vi "rsscope_core_global.vi"() -> ()   [LabVIEW 2014] (continued)
"Supported Models"="", "Instrument Options"="", "Flags"=0, "Help"="Starts the measurement.\n\nAvailable Repeated Capabilities:\nNone\n\nRemote-control command(s):\nPOWer:DONRes:EXECute"}, {"Level"=3, "Class Only"=FALSE, "Identifier"="RSSCOPE_ATTR_POWER_DYNAMIC_ON_RESISTANCE_AVERAGE", "Descriptive Name"="Power Dynamic On Resistance Average", "Data Type"=3, "Command"="POW:DONR:AVG", "Access"=2, "Range Table"="", "Read Callback"="", "Write Callback"="", "Supported Models"="", "Instrument Options"="", "Flags"=0, "Help"="Enables/disables averaging.\n\nAvailable Repeated Capabilities:\nNone\n\nRemote-control command(s):\nPOWer:DONRes:AVG"}, {"Level"=3, "Class Only"=FALSE, "Identifier"="RSSCOPE_ATTR_POWER_DYNAMIC_ON_RESISTANCE_SCALING", "Descriptive Name"="Power Dynamic On Resistance Scaling", "Data Type"=0, "Command"="POW:DONR:AUTO", "Access"=2, "Range Table"="RsScope_rngPowerScaling", "Read Callback"="", "Write Callback"="", "Supported Models"="", "Instrument Options"="", "Flags"=0, "Help"="Selects the scaling for the display of the results.\n\nAvailable Repeated Capabilities:\nNone\n\nRemote-control command(s):\nPOWer:DONRes:AUTO"}, {"Level"=3, "Class Only"=FALSE, "Identifier"="RSSCOPE_ATTR_POWER_DYNAMIC_ON_RESISTANCE_ADD", "Descriptive Name"="Power Dynamic On Resistance Add To Report", "Data Type"=4, "Command"="POW:DONR:REP:ADD", "Access"=1, "Range Table"="", "Read Callback"="", "Write Callback"="", "Supported Models"="", "Instrument Options"="", "Flags"=0, "Help"="Adds the result to the report list.\n\nAvailable Repeated Capabilities:\nNone\n\nRemote-control command(s):\nPOWer:DONRes:REPort:ADD"}, {"Level"=3, "Class Only"=TRUE, "Identifier"="", "Descriptive Name"="Gate", "Data Type"=0, "Command"="", "Access"=0, "Range Table"="", "Read Callback"="", "Write Callback"="", "Supported Models"="", "Instrument Options"="", "Flags"=0, "Help"="Attributes with gate repeated capability."}, {"Level"=4, "Class Only"=FALSE, "Identifier"="RSSCOPE_ATTR_POWER_DYNAMIC_ON_RESISTANCE_GATE_START", "Descriptive Name"="Power Dynamic On Resistance Gate Start", "Data Type"=1, "Command"="POW:DONR:GATE{Gate}:START", "Access"=2, "Range Table"="", "Read Callback"="", "Write Callback"="", "Supported Models"="", "Instrument Options"="", "Flags"=0, "Help"="Start of the gate.\n\nAvailable Repeated Capabilities:\nGate: Gate1, Gate2, Gate3, Gate4, Gate5\r\n\nRemote-control command(s):\nPOWer:DONRes:GATE<m>:STARt"}, {"Level"=4, "Class Only"=FALSE, "Identifier"="RSSCOPE_ATTR_POWER_DYNAMIC_ON_RESISTANCE_GATE_STOP", "Descriptive Name"="Power Dynamic On Resistance Gate Stop", "Data Type"=1, "Command"="POW:DONR:GATE{Gate}:STOP", "Access"=2, "Range Table"="", "Read Callback"="", "Write Callback"="", "Supported Models"="", "Instrument Options"="", "Flags"=0, "Help"="Stop of the gate.\n\nAvailable Repeated Capabilities:\nGate: Gate1, Gate2, Gate3, Gate4, Gate5\r\n\nRemote-control command(s):\nPOWer:DONRes:GATE<m>STOP"}, {"Level"=3, "Class Only"=TRUE, "Identifier"="", "Descriptive Name"="Results", "Data Type"=0, "Command"="", "Access"=0, "Range Table"="", "Read Callback"="", "Write Callback"="", "Supported Models"="", "Instrument Options"="", "Flags"=0, "Help"="Results of dynamic on resistance measurement"}, {"Level"=4, "Class Only"=FALSE, "Identifier"="RSSCOPE_ATTR_POWER_DYNAMIC_ON_RESISTANCE_RESULT", "Descriptive Name"="Power Dynamic On Resistance Result", "Data Type"=1, "Command"="POW:DONR:RES:RES?", "Access"=0, "Range Table"="", "Read Callback"="", "Write Callback"="", "Supported Models"="", "Instrument Options"="", "Flags"=0, "Help"="Returns the result of the measurement\n\nAvailable Repeated Capabilities:\nNone\n\nRemote-control command(s):\nPOWer:DONRes:RESult:RESistance?"}, {"Level"=2, "Class Only"=TRUE, "Identifier"="", "Descriptive Name"="Efficiency", "Data Type"=0, "Command"="", "Access"=0, "Range Table"="", "Read Callback"="", "Write Callback"="", "Supported Models"="", "Instrument Options"="", "Flags"=0, "Help"="Power efficiency measurement."}, {"Level"=3, "Class Only"=FALSE, "Identifier"="RSSCOPE_ATTR_START_POWER_EFFICIENCY_MEASUREMENT", "Descriptive Name"="Start Power Efficiency Measurement", "Data Type"=4, "Command"="POW:EFF:EXEC", "Access"=1, "Range Table"="", "Read Callback"="", "Write Callback"="", "Supported Models"="", "Instrument Options"="", "Flags"=0, "Help"="Starts the measurement.\n\nAvailable Repeated Capabilities:\nNone\n\nRemote-control command(s):\nPOWer:EFFiciency:EXECute"}, {"Level"=3, "Class Only"=FALSE, "Identifier"="RSSCOPE_ATTR_POWER_EFFICIENCY_SCALING", "Descriptive Name"="Power Efficiency Scaling", "Data Type"=0, "Command"="POW:EFF:AUTO", "Access"=2, "Range Table"="RsScope_rngPowerScaling", "Read Callback"="", "Write Callback"="", "Supported Models"="", "Instrument Options"="", "Flags"=0, "Help"="Selects the scaling for the display of the results.\n\nAvailable Repeated Capabilities:\nNone\n\nRemote-control command(s):\nPOWer:EFFiciency:AUTO"}, {"Level"=3, "Class Only"=FALSE, "Identifier"="RSSCOPE_ATTR_POWER_EFFICIENCY_ADD", "Descriptive Name"="Power Efficiency Add To Report", "Data Type"=4, "Command"="POW:EFF:REP:ADD", "Access"=1, "Range Table"="", "Read Callback"="", "Write Callback"="", "Supported Models"="", "Instrument Options"="", "Flags"=0, "Help"="Adds the result to the report list.\n\nAvailable Repeated Capabilities:\nNone\n\nRemote-control command(s):\nPOWer:EFFiciency:REPort:ADD"}, {"Level"=3, "Class Only"=TRUE, "Identifier"="", "Descriptive Name"="Results", "Data Type"=0, "Command"="", "Access"=0, "Range Table"="", "Read Callback"="", "Write Callback"="", "Supported Models"="", "Instrument Options"="", "Flags"=0, "Help"="Results of the measurement."}, {"Level"=2, "Class Only"=TRUE, "Identifier"="", "Descriptive Name"="Switchingloss", "Data Type"=0, "Command"="", "Access"=0, "Range Table"="", "Read Callback"="", "Write Callback"="", "Supported Models"="", "Instrument Options"="", "Flags"=0, "Help"="Switchingloss measurement"}, {"Level"=3, "Class Only"=FALSE, "Identifier"="RSSCOPE_ATTR_START_POWER_SWITCHINGLOSS_MEASUREMENT", "Descriptive Name"="Start Power Switchingloss Measurement", "Data Type"=4, "Command"="POW:SWIT:EXEC", "Access"=1, "Range Table"="", "Read Callback"="", "Write Callback"="", "Supported Models"="", "Instrument Options"="", "Flags"=0, "Help"="Starts the measurement.\n\nAvailable Repeated Capabilities:\nNone\n\nRemote-control command(s):\nPOWer:SWITching:EXECute"}, {"Level"=3, "Class Only"=FALSE, "Identifier"="RSSCOPE_ATTR_POWER_SWITCHINGLOSS_TON_STATE", "Descriptive Name"="Power Switchingloss Turn On State", "Data Type"=3, "Command"="POW:SWIT:TON", "Access"=2, "Range Table"="", "Read Callback"="", "Write Callback"="", "Supported Models"="", "Instrument Options"="", "Flags"=0, "Help"="Enables the measurement during the Turn On period.\n\nAvailable Repeated Capabilities:\nNone\n\nRemote-control command(s):\nPOWer:SWITching:TON"}, {"Level"=3, "Class Only"=FALSE, "Identifier"="RSSCOPE_ATTR_POWER_SWITCHINGLOSS_TOF_STATE", "Descriptive Name"="Power Switchingloss Turn Off State", "Data Type"=3, "Command"="POW:SWIT:TOFF", "Access"=2, "Range Table"="", "Read Callback"="", "Write Callback"="", "Supported Models"="", "Instrument Options"="", "Flags"=0, "Help"="Enables the measurement during the Turn Off period.\n\nAvailable Repeated Capabilities:\nNone\n\nRemote-control command(s):\nPOWer:SWITching:TOFF"}, {"Level"=3, "Class Only"=FALSE, "Identifier"="RSSCOPE_ATTR_POWER_SWITCHINGLOSS_CONDUCTION_STATE", "Descriptive Name"="Power Switchingloss Conduction State", "Data Type"=3, "Command"="POW:SWIT:COND", "Access"=2, "Range Table"="", "Read Callback"="", "Write Callback"="", "Supported Models"="", "Instrument Options"="", "Flags"=0, "Help"="Enables the measurement during the Conduction period.\n\nAvailable Repeated Capabilities:\nNone\n\nRemote-control command(s):\nPOWer:SWITching:COND"}, {"Level"=3, "Class Only"=FALSE, "Identifier"="RSSCOPE_ATTR_POWER_SWITCHINGLOSS_NON_CONDUCTION_STATE", "Descriptive Name"="Power Switchingloss Non Conduction State", "Data Type"=3, "Command"="POW:SWIT:NCON", "Access"=2, "Range Table"="", "Read Callback"="", "Write Callback"="", "Supported Models"="", "Instrument Options"="", "Flags"=0, "Help"="Enables the measurement during the Non Conduction period.\n\nAvailable Repeated Capabilities:\nNone\n\nRemote-control command(s):\nPOWer:SWITching:NCON"}, {"Level"=3, "Class Only"=FALSE, "Identifier"="RSSCOPE_ATTR_POWER_SWITCHINGLOSS_TOTAL_STATE", "Descriptive Name"="Power Switchingloss Total State", "Data Type"=3, "Command"="POW:SWIT:TOT", "Access"=2, "Range Table"="", "Read Callback"="", "Write Callback"="", "Supported Models"="", "Instrument Options"="", "Flags"=0, "Help"="Enables the measurement of the total period\n\nAvailable Repeated Capabilities:\nNone\n\nRemote-control command(s):\nPOWer:SWITching:TOTal"}, {"Level"=3, "Class Only"=FALSE, "Identifier"="RSSCOPE_ATTR_POWER_SWITCHINGLOSS_SWITCHING_FREQUENCY_STATE", "Descriptive Name"="Power Switchingloss Switching Frequency State", "Data Type"=3, "Command"="POW:SWIT:SWIT", "Access"=2, "Range Table"="", "Read Callback"="", "Write Callback"="", "Supported Models"="", "Instrument Options"="", "Flags"=0, "Help"="Enables the measurements of the switching frequency\n\nAvailable Repeated Capabilities:\nNone\n\nRemote-control command(s):\nPOWer:SWITching:SWIT"}, {"Level"=3, "Class Only"=FALSE, "Identifier"="RSSCOPE_ATTR_POWER_SWITCHINGLOSS_SWITCHING_FREQUENCY_VALUE", "Descriptive Name"="Power Switchingloss Switching Frequency Value", "Data Type"=1, "Command"="POW:SWIT:SWIF", "Access"=2, "Range Table"="RsScope_rngPowerSwitchinglossSwitchingFrequencyValue", "Read Callback"="", "Write Callback"="", "Supported Models"="", "Instrument Options"="", "Flags"=0, "Help"="Sets the switching frequency\n\nAvailable Repeated Capabilities:\nNone\n\nRemote-control command(s):\nPOWer:SWITching:SWIFrequency"}, {"Level"=3, "Class Only"=FALSE, "Identifier"="RSSCOPE_ATTR_POWER_SWITCHINGLOSS_SCALING", "Descriptive Name"="Power Switchingloss Scaling", "Data Type"=0, "Command"="POW:SWIT:AUTO", "Access"=2, "Range Table"="RsScope_rngPowerScaling", "Read Callback"="", "Write Callback"="", "Supported Models"="", "Instrument Options"="", "Flags"=0, "Help"="Selects the scaling for the display of the results.\n\nAvailable Repeated Capabilities:\nNone\n\nRemote-control command(s):\nPOWer:SWITching:AUTO"}, {"Level"=3, "Class Only"=FALSE, "Identifier"="RSSCOPE_ATTR_POWER_SWITCHINGLOSS_ADD", "Descriptive Name"="Power Switchingloss Add To Report", "Data Type"=4, "Command"="POW:SWIT:REP:ADD", "Access"=1, "Range Table"="", "Read Callback"="", "Write Callback"="", "Supported Models"="", "Instrument Options"="", "Flags"=0, "Help"="Adds the result to the report list.\n\nAvailable Repeated Capabilities:\nNone\n\nRemote-control command(s):\nPOWer:SWITching:REPort:ADD"}, {"Level"=3, "Class Only"=TRUE, "Identifier"="", "Descriptive Name"="Gate", "Data Type"=0, "Command"="", "Access"=0, "Range Table"="", "Read Callback"="", "Write Callback"="", "Supported Models"="", "Instrument Options"="", "Flags"=0, "Help"="Configures gate."}, {"Level"=4, "Class Only"=FALSE, "Identifier"="RSSCOPE_ATTR_POWER_SWITCHINGLOSS_GATE_CONDUCTION_START", "Descriptive Name"="Power Switchingloss Gate Conduction Start", "Data Type"=1, "Command"="POW:SWIT:GATE:COND:STAR", "Access"=2, "Range Table"="", "Read Callback"="", "Write Callback"="", "Supported Models"="", "Instrument Options"="", "Flags"=0, "Help"="Start of the gate.\n\nAvailable Repeated Capabilities:\nNone\n\nRemote-control command(s):\nPOWer:SWITching:GATE:COND:STARt"}, {"Level"=4, "Class Only"=FALSE, "Identifier"="RSSCOPE_ATTR_POWER_SWITCHINGLOSS_GATE_CONDUCTION_STOP", "Descriptive Name"="Power Switchingloss Gate Conduction Stop", "Data Type"=1, "Command"="POW:SWIT:GATE:COND:STOP", "Access"=2, "Range Table"="", "Read Callback"="", "Write Callback"="", "Supported Models"="", "Instrument Options"="", "Flags"=0, "Help"="Stop of the gate.\n\nAvailable Repeated Capabilities:\nNone\n\nRemote-control command(s):\nPOWer:SWITching:GATE:COND:STOP"}, {"Level"=4, "Class Only"=FALSE, "Identifier"="RSSCOPE_ATTR_POWER_SWITCHINGLOSS_GATE_NO_CONDUCTION_START", "Descriptive Name"="Power Switchingloss Gate No Conduction Start", "Data Type"=1, "Command"="POW:SWIT:GATE:NCON:STAR", "Access"=2, "Range Table"="", "Read Callback"="", "Write Callback"="", "Supported Models"="", "Instrument Options"="", "Flags"=0, "Help"="Start of the gate.\n\nAvailable Repeated Capabilities:\nNone\n\nRemote-control command(s):\nPOWer:SWITching:GATE:NCON:STARt"}, {"Level"=4, "Class Only"=FALSE, "Identifier"="RSSCOPE_ATTR_POWER_SWITCHINGLOSS_GATE_NO_CONDUCTION_STOP", "Descriptive Name"="Power Switchingloss Gate No Conduction Stop", "Data Type"=1, "Command"="POW:SWIT:GATE:NCON:STOP", "Access"=2, "Range Table"="", "Read Callback"="", "Write Callback"="", "Supported Models"="", "Instrument Options"="", "Flags"=0, "Help"="Stop of the gate.\n\nAvailable Repeated Capabilities:\nNone\n\nRemote-control command(s):\nPOWer:SWITching:GATE:NCON:STOP"}, {"Level"=4, "Class Only"=FALSE, "Identifier"="RSSCOPE_ATTR_POWER_SWITCHINGLOSS_GATE_TURN_ON_START", "Descriptive Name"="Power Switchingloss Gate Turn On Start", "Data Type"=1, "Command"="POW:SWIT:GATE:TON:STAR", "Access"=2, "Range Table"="", "Read Callback"="", "Write Callback"="", "Supported Models"="", "Instrument Options"="", "Flags"=0, "Help"="Start of the gate.\n\nAvailable Repeated Capabilities:\nNone\n\nRemote-control command(s):\nPOWer:SWITching:GATE:TON:STARt"}, {"Level"=4, "Class Only"=FALSE, "Identifier"="RSSCOPE_ATTR_POWER_SWITCHINGLOSS_GATE_TURN_ON_STOP", "Descriptive Name"="Power Switchingloss Gate Turn On Stop", "Data Type"=1, "Command"="POW:SWIT:GATE:TON:STOP", "Access"=2, "Range Table"="", "Read Callback"="", "Write Callback"="", "Supported Models"="", "Instrument Options"="", "Flags"=0, "Help"="Stop of the gate.\n\nAvailable Repeated Capabilities:\nNone\n\nRemote-control command(s):\nPOWer:SWITching:GATE:TON:STOP"}, {"Level"=4, "Class Only"=FALSE, "Identifier"="RSSCOPE_ATTR_POWER_SWITCHINGLOSS_GATE_TURN_OFF_START", "Descriptive Name"="Power Switchingloss Gate Turn Off Start", "Data Type"=1, "Command"="POW:SWIT:GATE:TOFF:STAR", "Access"=2, "Range Table"="", "Read Callback"="", "Write Callback"="", "Supported Models"="", "Instrument Options"="", "Flags"=0, "Help"="Start of the gate.\n\nAvailable Repeated Capabilities:\nNone\n\nRemote-control command(s):\nPOWer:SWITching:GATE:TOFF:STARt"}, {"Level"=4, "Class Only"=FALSE, "Identifier"="RSSCOPE_ATTR_POWER_SWITCHINGLOSS_GATE_TURN_OFF_STOP", "Descriptive Name"="Power Switchingloss Gate Turn Off Stop", "Data Type"=1, "Command"="POW:SWIT:GATE:TOFF:STOP", "Access"=2, "Range Table"="", "Read Callback"="", "Write Callback"="", "Supported Models"="", "Instrument Options"="", "Flags"=0, "Help"="Stop of the gate.\n\nAvailable Repeated Capabilities:\nNone\n\nRemote-control command(s):\nPOWer:SWITching:GATE:TOFF:STOP"}, {"Level"=3, "Class Only"=TRUE, "Identifier"="", "Descriptive Name"="Results", "Data Type"=0, "Command"="", "Access"=0, "Range Table"="", "Read Callback"="", "Write Callback"="", "Supported Models"="", "Instrument Options"="", "Flags"=0, "Help"="Results of the measurement."}, {"Level"=2, "Class Only"=TRUE, "Identifier"="", "Descriptive Name"="On Off Measurement", "Data Type"=0, "Command"="", "Access"=0, "Range Table"="", "Read Callback"="", "Write Callback"="", "Supported Models"="", "Instrument Options"="", "Flags"=0, "Help"="Power on/off measurement."}, {"Level"=3, "Class Only"=FALSE, "Identifier"="RSSCOPE_ATTR_START_POWER_ON_OFF_MEASUREMENT", "Descriptive Name"="Start Power On Off Measurement", "Data Type"=4, "Command"="POW:ONOF:EXEC", "Access"=1, "Range Table"="", "Read Callback"="", "Write Callback"="", "Supported Models"="", "Instrument Options"="", "Flags"=0, "Help"="Starts the measurement.\n\nAvailable Repeated Capabilities:\nNone\n\nRemote-control command(s):\nPOWer:ONOFf:EXECute"}, {"Level"=3, "Class Only"=FALSE, "Identifier"="RSSCOPE_ATTR_POWER_ON_OFF_TYPE", "Descriptive Name"="On Off Type", "Data Type"=0, "Command"="POW:ONOF:TYPE", "Access"=2, "Range Table"="RsScope_rngOnOffType", "Read Callback"="", "Write Callback"="", "Supported Models"="", "Instrument Options"="", "Flags"=0, "Help"="Selects the turn on or the turn off measurement.\n\nAvailable Repeated Capabilities:\nNone\n\nRemote-control command(s):\nPOWer:ONOFf:TYPE"}, {"Level"=3, "Class Only"=FALSE, "Identifier"="RSSCOPE_ATTR_POWER_ON_OFF_TIME", "Descriptive Name"="On Off Time", "Data Type"=1, "Command"="POW:ONOF:TIME", "Access"=2, "Range Table"="RsScope_rngOnOffTime", "Read Callback"="", "Write Callback"="", "Supported Models"="", "Instrument Options"="", "Flags"=0, "Help"="Sets the time the start of the measurement of the turn off time is delay with, after the trigger point.\n\nAvailable Repeated Capabilities:\nNone\n\nRemote-control command(s):\nPOWer:ONOFf:TIME"}, {"Level"=3, "Class Only"=FALSE, "Identifier"="RSSCOPE_ATTR_POWER_ON_STEADY_STATE_LEVEL", "Descriptive Name"="On Steady State Level", "Data Type"=1, "Command"="POW:ONOF:DSON", "Access"=2, "Range Table"="RsScope_rngOnOffSteadyStateLevel", "Read Callback"="", "Write Callback"="", "Supported Models"="", "Instrument Options"="", "Flags"=0, "Help"="Sets the percentage of the steady state level of the DC output that has to be reached.\n\nAvailable Repeated Capabilities:\nNone\n\nRemote-control command(s):\nPOWer:ONOFf:DSON"}, {"Level"=3, "Class Only"=FALSE, "Identifier"="RSSCOPE_ATTR_POWER_OFF_STEADY_STATE_LEVEL", "Descriptive Name"="Off Steady State Level", "Data Type"=1, "Command"="POW:ONOF:DSOF", "Access"=2, "Range Table"="RsScope_rngOnOffSteadyStateLevel", "Read Callback"="", "Write Callback"="", "Supported Models"="", "Instrument Options"="", "Flags"=0, "Help"="Sets the percentage of the steady state level of the DC output that has to be reached.\n\nAvailable Repeated Capabilities:\nNone\n\nRemote-control command(s):\nPOWer:ONOFf:DSOFf"}, {"Level"=3, "Class Only"=FALSE, "Identifier"="RSSCOPE_ATTR_POWER_ON_TRIGGER_LEVEL", "Descriptive Name"="On Trigger Level", "Data Type"=1, "Command"="POW:ONOF:ATON", "Access"=2, "Range Table"="RsScope_rngOnOffTriggerLevel", "Read Callback"="", "Write Callback"="", "Supported Models"="", "Instrument Options"="", "Flags"=0, "Help"="Triggers the beginning of the measurements at the moment the AC voltage reaches the set value.\n\nAvailable Repeated Capabilities:\nNone\n\nRemote-control command(s):\nPOWer:ONOFf:ATON"}, {"Level"=3, "Class Only"=FALSE, "Identifier"="RSSCOPE_ATTR_POWER_ON_TRIGGER_LEVEL_DC", "Descriptive Name"="On Trigger Level DC", "Data Type"=1, "Command"="POW:ONOF:DTON", "Access"=2, "Range Table"="RsScope_rngOnOffTriggerLevel", "Read Callback"="", "Write Callback"="", "Supported Models"="", "Instrument Options"="", "Flags"=0, "Help"="Triggers the beginning of the measurements at the moment the DC input voltage reaches the set value.\n\nAvailable Repeated Capabilities:\nNone\n\nRemote-control command(s):\nPOWer:ONOFf:DTON"}, {"Level"=3, "Class Only"=FALSE, "Identifier"="RSSCOPE_ATTR_POWER_OFF_TRIGGER_LEVEL", "Descriptive Name"="Off Trigger Level", "Data Type"=1, "Command"="POW:ONOF:ATOF", "Access"=2, "Range Table"="RsScope_rngOnOffTriggerLevel", "Read Callback"="", "Write Callback"="", "Supported Models"="", "Instrument Options"="", "Flags"=0, "Help"="Triggers the beginning of the measurements at the moment the AC voltage reaches the set value.\n\nAvailable Repeated Capabilities:\nNone\n\nRemote-control command(s):\nPOWer:ONOFf:ATOFf"}, {"Level"=3, "Class Only"=FALSE, "Identifier"="RSSCOPE_ATTR_POWER_OFF_TRIGGER_LEVEL_DC", "Descriptive Name"="Off Trigger Level DC", "Data Type"=1, "Command"="POW:ONOF:DTOF", "Access"=2, "Range Table"="RsScope_rngOnOffTriggerLevel", "Read Callback"="", "Write Callback"="", "Supported Models"="", "Instrument Options"="", "Flags"=0, "Help"="Triggers the beginning of the measurements at the moment the DC input voltage reaches the set value.\n\nAvailable Repeated Capabilities:\nNone\n\nRemote-control command(s):\nPOWer:ONOFf:DTOFf"}, {"Level"=3, "Class Only"=FALSE, "Identifier"="RSSCOPE_ATTR_POWER_ON_OFF_ADD", "Descriptive Name"="On Off Add To Report", "Data Type"=4, "Command"="POW:ONOF:REP:ADD", "Access"=1, "Range Table"="", "Read Callback"="", "Write Callback"="", "Supported Models"="", "Instrument Options"="", "Flags"=0, "Help"="Adds the result to the report list.\n\nAvailable Repeated Capabilities:\nNone\n\nRemote-control command(s):\nPOWer:ONOFf:REPort:ADD"}, {"Level"=3, "Class Only"=FALSE, "Identifier"="RSSCOPE_ATTR_POWER_ON_OFF_INPUT_TYPE", "Descriptive Name"="On Off Input Type", "Data Type"=0, "Command"="POW:ONOF:INP", "Access"=2, "Range Table"="rsscope_rngOnOffInputType", "Read Callback"="", "Write Callback"="", "Supported Models"="", "Instrument Options"="", "Flags"=0, "Help"="Sets the input type.\n\nAvailable Repeated Capabilities:\nNone\n\nRemote-control command(s):\nPOWer:ONOFf:INPut"}, {"Level"=3, "Class Only"=TRUE, "Identifier"="", "Descriptive Name"="Results", "Data Type"=0, "Command"="", "Access"=0, "Range Table"="", "Read Callback"="", "Write Callback"="", "Supported Models"="", "Instrument Options"="", "Flags"=0, "Help"="Measurement result"}, {"Level"=4, "Class Only"=FALSE, "Identifier"="RSSCOPE_ATTR_POWER_ON_RESULT", "Descriptive Name"="Turn On Result", "Data Type"=1, "Command"="POW:ONOF:RES:TON?", "Access"=0, "Range Table"="", "Read Callback"="", "Write Callback"="", "Supported Models"="", "Instrument Options"="", "Flags"=0, "Help"="Returns the turn On time\n\nAvailable Repeated Capabilities:\nNone\n\nRemote-control command(s):\nPOWer:ONOFf:RESult:TON?"}, {"Level"=4, "Class Only"=FALSE, "Identifier"="RSSCOPE_ATTR_POWER_OFF_RESULT", "Descriptive Name"="Turn Off Result", "Data Type"=1, "Command"="POW:ONOF:RES:TOFF?", "Access"=0, "Range Table"="", "Read Callback"="", "Write Callback"="", "Supported Models"="", "Instrument Options"="", "Flags"=0, "Help"="Returns the turn Off time\n\nAvailable Repeated Capabilities:\nNone\n\nRemote-control command(s):\nPOWer:ONOFf:RESult:TOFF?"}, {"Level"=2, "Class Only"=TRUE, "Identifier"="", "Descriptive Name"="Transient Response", "Data Type"=0, "Command"="", "Access"=0, "Range Table"="", "Read Callback"="", "Write Callback"="", "Supported Models"="", "Instrument Options"="", "Flags"=0, "Help"="Measures the response of a system to a change from equilibrium. This response is described by different properties like the rise time, the overshoot, the settling time, the peak time and the delay time"}, {"Level"=3, "Class Only"=FALSE, "Identifier"="RSSCOPE_ATTR_START_POWER_TRANSIENT_RESPONSE_MEASUREMENT", "Descriptive Name"="Start Power Transient Response Measurement", "Data Type"=4, "Command"="POW:TRAN:EXEC", "Access"=1, "Range Table"="", "Read Callback"="", "Write Callback"="", "Supported Models"="", "Instrument Options"="", "Flags"=0, "Help"="Starts the transient response measurement.\n\nAvailable Repeated Capabilities:\nNone\n\nRemote-control command(s):\nPOWer:TRANsient:EXECute"}, {"Level"=3, "Class Only"=FALSE, "Identifier"="RSSCOPE_ATTR_POWER_TRANSIENT_RESPONSE_INPUT_STATE", "Descriptive Name"="Transient Response Input State", "Data Type"=3, "Command"="POW:TRAN:INP", "Access"=2, "Range Table"="", "Read Callback"="", "Write Callback"="", "Supported Models"="", "Instrument Options"="", "Flags"=0, "Help"="Activates or deactivates the input voltage.\n\nAvailable Repeated Capabilities:\nNone\n\nRemote-control command(s):\nPOWer:TRANsient:INPut"}, {"Level"=3, "Class Only"=FALSE, "Identifier"="RSSCOPE_ATTR_POWER_TRANSIENT_RESPONSE_TRIGGER_SOURCE", "Descriptive Name"="Transient Response Trigger Source", "Data Type"=0, "Command"="POW:TRAN:TRGC", "Access"=2, "Range Table"="RsScope_rngTransientResponseTriggerSource", "Read Callback"="", "Write Callback"="", "Supported Models"="", "Instrument Options"="", "Flags"=0, "Help"="Sets the source channel of the trigger.\n\nAvailable Repeated Capabilities:\nNone\n\nRemote-control command(s):\nPOWer:TRANsient:TRGChannel"}, {"Level"=3, "Class Only"=FALSE, "Identifier"="RSSCOPE_ATTR_POWER_TRANSIENT_RESPONSE_TRIGGER_LEVEL", "Descriptive Name"="Transient Response Trigger Level", "Data Type"=1, "Command"="POW:TRAN:TRGL", "Access"=2, "Range Table"="rsscope_rngTriggerLevel", "Read Callback"="", "Write Callback"="", "Supported Models"="", "Instrument Options"="", "Flags"=0, "Help"="Sets the trigger level.\n\nAvailable Repeated Capabilities:\nNone\n\nRemote-control command(s):\nPOWer:TRANsient:TRGLevel"}, {"Level"=3, "Class Only"=FALSE, "Identifier"="RSSCOPE_ATTR_POWER_TRANSIENT_RESPONSE_TRIGGER_SLOPE", "Descriptive Name"="Transient Response Trigger Slope", "Data Type"=0, "Command"="POW:TRAN:TRGS", "Access"=2, "Range Table"="rsscope_rngTriggerSlope", "Read Callback"="", "Write Callback"="", "Supported Models"="", "Instrument Options"="", "Flags"=0, "Help"="Sets the edge type for the trigger event.\n\nAvailable Repeated Capabilities:\nNone\n\nRemote-control command(s):\nPOWer:TRANsient:TRGSlope"}, {"Level"=3, "Class Only"=FALSE, "Identifier"="RSSCOPE_ATTR_POWER_TRANSIENT_RESPONSE_TUBE_TOLERANCE", "Descriptive Name"="Transient Response Tube Tolerance", "Data Type"=0, "Command"="POW:TRAN:HYST", "Access"=2, "Range Table"="RsScope_rngTransientResponseTubeTolerance", "Read Callback"="", "Write Callback"="", "Supported Models"="", "Instrument Options"="", "Flags"=0, "Help"="Specifies a tolerated error band for the signal level\n\nAvailable Repeated Capabilities:\nNone\n\nRemote-control command(s):\nPOWer:TRANsient:HYSTeresis"}, {"Level"=3, "Class Only"=FALSE, "Identifier"="RSSCOPE_ATTR_POWER_TRANSIENT_RESPONSE_SIGNAL_HIGH", "Descriptive Name"="Transient Response Signal High", "Data Type"=1, "Command"="POW:TRAN:SIGH", "Access"=2, "Range Table"="RsScope_rngTransientResponseSignal", "Read Callback"="", "Write Callback"="", "Supported Models"="", "Instrument Options"="", "Flags"=0, "Help"="Sets the expected signal high voltage value.\n\nAvailable Repeated Capabilities:\nNone\n\nRemote-control command(s):\nPOWer:TRANsient:SIGHigh"}, {"Level"=3, "Class Only"=FALSE, "Identifier"="RSSCOPE_ATTR_POWER_TRANSIENT_RESPONSE_SIGNAL_LOW", "Descriptive Name"="Transient Response Signal Low", "Data Type"=1, "Command"="POW:TRAN:SIGL", "Access"=2, "Range Table"="RsScope_rngTransientResponseSignal", "Read Callback"="", "Write Callback"="", "Supported Models"="", "Instrument Options"="", "Flags"=0, "Help"="Sets the expected signal low voltage value.\n\nAvailable Repeated Capabilities:\nNone\n\nRemote-control command(s):\nPOWer:TRANsient:SIGLow"}, {"Level"=3, "Class Only"=FALSE, "Identifier"="RSSCOPE_ATTR_POWER_TRANSIENT_RESPONSE_FREQUENCY", "Descriptive Name"="Transient Response Frequency", "Data Type"=1, "Command"="POW:TRAN:FREQ", "Access"=2, "Range Table"="RsScope_rngPowerSwitchingFrequency", "Read Callback"="", "Write Callback"="", "Supported Models"="", "Instrument Options"="", "Flags"=0, "Help"="Sets the SMPS switching frequency.\n\nAvailable Repeated Capabilities:\nNone\n\nRemote-control command(s):\nPOWer:TRANsient:FREQuency"}, {"Level"=3, "Class Only"=FALSE, "Identifier"="RSSCOPE_ATTR_POWER_TRANSIENT_RESPONSE_SCALING", "Descriptive Name"="Power Transient Response Scaling", "Data Type"=0, "Command"="POW:TRAN:AUT", "Access"=2, "Range Table"="RsScope_rngPowerScaling", "Read Callback"="", "Write Callback"="", "Supported Models"="", "Instrument Options"="", "Flags"=0, "Help"="Selects the scaling for the display of the results.\n\nAvailable Repeated Capabilities:\nNone\n\nRemote-control command(s):\nPOWer:TRANsient:AUToscale"}, {"Level"=3, "Class Only"=FALSE, "Identifier"="RSSCOPE_ATTR_POWER_TRANSIENT_RESPONSE_ADD", "Descriptive Name"="Transient Response Add To Report", "Data Type"=4, "Command"="POWer:TRANsient:REPort:ADD", "Access"=1, "Range Table"="", "Read Callback"="", "Write Callback"="", "Supported Models"="", "Instrument Options"="", "Flags"=0, "Help"="Adds the result to the report list.\n\nAvailable Repeated Capabilities:\nNone\n\nRemote-control command(s):\nPOWer:TRANsient:REPort:ADD"}, {"Level"=3, "Class Only"=TRUE, "Identifier"="", "Descriptive Name"="Results", "Data Type"=0, "Command"="", "Access"=0, "Range Table"="", "Read Callback"="", "Write Callback"="", "Supported Models"="", "Instrument Options"="", "Flags"=0, "Help"="Returns transient response results."}, {"Level"=1, "Class Only"=TRUE, "Identifier"="", "Descriptive Name"="Deembedding", "Data Type"=0, "Command"="", "Access"=0, "Range Table"="", "Read Callback"="", "Write Callback"="", "Supported Models"="", "Instrument Options"="", "Flags"=0, "Help"="Deembedding (Option R&S RTO-K121)"}, {"Level"=2, "Class Only"=FALSE, "Identifier"="RSSCOPE_ATTR_DEEMBEDDING_STATE", "Descriptive Name"="Deembedding State", "Data Type"=3, "Command"="DEEM{Channel}", "Access"=2, "Range Table"="", "Read Callback"="", "Write Callback"="", "Supported Models"="", "Instrument Options"="K121", "Flags"=0, "Help"="Activates the deembedding - the correction of parasitic effects of the measurement setup on the measured signal.\n\nAvailable Repeated Capabilities:\nChannel: CH1, CH2, CH3, CH4, CHExt\r\n\nRemote-control command(s):\nDEEMbedding<m>[:STATe]"}, {"Level"=2, "Class Only"=FALSE, "Identifier"="RSSCOPE_ATTR_DEEMBEDDING_EFFECTIVE_BANDWIDTH", "Descriptive Name"="Deembedding Effective Bandwidth", "Data Type"=1, "Command"="DEEM{Channel}:BAND", "Access"=2, "Range Table"="RsScope_rngDeembeddingEffectiveBandwidth", "Read Callback"="", "Write Callback"="", "Supported Models"="", "Instrument Options"="K121", "Flags"=0, "Help"="Sets the maximum bandwidth until which the signal is corrected. This maximum value is the minimum bandwidth value of probe, probe tip and oscilloscope bandwidth, and can not be higher than the highest frequency in a used S-parameter file.\n\nAvailable Repeated Capabilities:\nChannel: CH1, CH2, CH3, CH4, CHExt\r\n\nRemote-control command(s):\nDEEMbedding<m>:BANDwidth"}, {"Level"=2, "Class Only"=FALSE, "Identifier"="RSSCOPE_ATTR_DEEMBEDDING_DELAY_COMPENSATION", "Descriptive Name"="Deembedding Delay Compensation", "Data Type"=3, "Command"="DEEM{Channel}:CMPD", "Access"=2, "Range Table"="", "Read Callback"="", "Write Callback"="", "Supported Models"="", "Instrument Options"="K121", "Flags"=0, "Help"="Enables the compensation for the group delay of the complete measurement setup. If enabled, the calibration time reference point is the start point of the measurement setup. If disabled, the calibration time reference point is the oscilloscope&apos;s channel input.\n\nAvailable Repeated Capabilities:\nChannel: CH1, CH2, CH3, CH4, CHExt\r\n\nRemote-control command(s):\nDEEMbedding<m>:CMPDelay"}, {"Level"=2, "Class Only"=FALSE, "Identifier"="RSSCOPE_ATTR_DEEMBEDDING_REALTIME_ENABLED", "Descriptive Name"="Deembedding Realtime Enabled", "Data Type"=3, "Command"="DEEM{Channel}:REAL", "Access"=2, "Range Table"="", "Read Callback"="", "Write Callback"="", "Supported Models"="", "Instrument Options"="K122", "Flags"=0, "Help"="If ON, the deembedding calculation is done by the hardware in real time. You can trigger on the corrected signal, and the acquisition rate remains unchanged.\nIf OFF, the deembedding calculation is done by software. This method is slower, therefore, triggering on the corrected signal is not possible.\n\nAvailable Repeated Capabilities:\nChannel: CH1, CH2, CH3, CH4, CHExt\r\n\nRemote-control command(s):\nDEEMbedding<m>:REALtime"}, {"Level"=2, "Class Only"=FALSE, "Identifier"="RSSCOPE_ATTR_DEEMBEDDING_REMOVE_COMPONENT", "Descriptive Name"="Deembedding Remove Component", "Data Type"=0, "Command"="DEEM{Channel}:REM", "Access"=2, "Range Table"="", "Read Callback"="", "Write Callback"="", "Supported Models"="", "Instrument Options"="K121", "Flags"=0, "Help"="Deletes the component with the indicated index from the measurement setup.\n\nAvailable Repeated Capabilities:\nChannel: CH1, CH2, CH3, CH4, CHExt\r\n\nRemote-control command(s):\nDEEMbedding<m>:REMove"}, {"Level"=2, "Class Only"=FALSE, "Identifier"="RSSCOPE_ATTR_DEEMBEDDING_COMPONENT_COUNT", "Descriptive Name"="Deembedding Component Count", "Data Type"=0, "Command"="DEEM{Channel}:CCO?", "Access"=0, "Range Table"="", "Read Callback"="", "Write Callback"="", "Supported Models"="", "Instrument Options"="K121", "Flags"=0, "Help"="Returns the total number of components in the measurement setup, including disabled components.\n\nAvailable Repeated Capabilities:\nChannel: CH1, CH2, CH3, CH4, CHExt\r\n\nRemote-control command(s):\nDEEMbedding<m>:CCOunt?"}, {"Level"=2, "Class Only"=FALSE, "Identifier"="RSSCOPE_ATTR_DEEMBEDDING_SETTINGS_FILE_NAME", "Descriptive Name"="Deembedding Settings File Name", "Data Type"=2, "Command"="DEEM{Channel}:NAME", "Access"=2, "Range Table"="", "Read Callback"="", "Write Callback"="", "Supported Models"="", "Instrument Options"="K121", "Flags"=0, "Help"="Sets the file name, file format and path of the deembedding setup file. The file format is always .xml.\n\nAvailable Repeated Capabilities:\nChannel: CH1, CH2, CH3, CH4, CHExt\r\n\nRemote-control command(s):\nDEEMbedding<m>:NAME"}, {"Level"=2, "Class Only"=FALSE, "Identifier"="RSSCOPE_ATTR_DEEMBEDDING_SAVE_SETTINGS", "Descriptive Name"="Deembedding Save Settings", "Data Type"=4, "Command"="DEEM{Channel}:SAVE", "Access"=1, "Range Table"="", "Read Callback"="", "Write Callback"="", "Supported Models"="", "Instrument Options"="K121", "Flags"=0, "Help"="Saves the deembedding configuration to the file specified with RSSCOPE_ATTR_DEEMBEDDING_SETTINGS_FILE_NAME.\n\nAvailable Repeated Capabilities:\nChannel: CH1, CH2, CH3, CH4, CHExt\r\n\nRemote-control command(s):\nDEEMbedding<m>:SAVE"}, {"Level"=2, "Class Only"=FALSE, "Identifier"="RSSCOPE_ATTR_DEEMBEDDING_LOAD_SETTINGS", "Descriptive Name"="Deembedding Load Settings", "Data Type"=4, "Command"="DEEM{Channel}:OPEN", "Access"=1, "Range Table"="", "Read Callback"="", "Write Callback"="", "Supported Models"="", "Instrument Options"="K121", "Flags"=0, "Help"="Opens and loads the deembedding configuration from the file specified with RSSCOPE_ATTR_DEEMBEDDING_SETTINGS_FILE_NAME.\n\nAvailable Repeated Capabilities:\nChannel: CH1, CH2, CH3, CH4, CHExt\r\n\nRemote-control command(s):\nDEEMbedding<m>:OPEN"}, {"Level"=2, "Class Only"=FALSE, "Identifier"="RSSCOPE_ATTR_DEEMBEDDING_DELETE_SETTINGS", "Descriptive Name"="Deembedding Delete Settings", "Data Type"=4, "Command"="DEEM{Channel}:DEL", "Access"=1, "Range Table"="", "Read Callback"="", "Write Callback"="", "Supported Models"="", "Instrument Options"="K121", "Flags"=0, "Help"="Deletes the deembedding configuration file specified with RSSCOPE_ATTR_DEEMBEDDING_SETTINGS_FILE_NAME.\n\nAvailable Repeated Capabilities:\nChannel: CH1, CH2, CH3, CH4, CHExt\r\n\nRemote-control command(s):\nDEEMbedding<m>:DELete"}, {"Level"=2, "Class Only"=FALSE, "Identifier"="RSSCOPE_ATTR_DEEMBEDDING_PRESET", "Descriptive Name"="Deembedding Preset", "Data Type"=4, "Command"="DEEM{Channel}:PRES", "Access"=1, "Range Table"="", "Read Callback"="", "Write Callback"="", "Supported Models"="", "Instrument Options"="K121", "Flags"=0, "Help"="Sets the complete deembedding configuration to the default values.\n\nAvailable Repeated Capabilities:\nChannel: CH1, CH2, CH3, CH4, CHExt\r\n\nRemote-control command(s):\nDEEMbedding<m>:PRESet"}, {"Level"=2, "Class Only"=FALSE, "Identifier"="RSSCOPE_ATTR_DEEMBEDDING_SELECTED_COMPONENT", "Descriptive Name"="Deembedding Selected Component", "Data Type"=0, "Command"="", "Access"=2, "Range Table"="", "Read Callback"="", "Write Callback"="", "Supported Models"="", "Instrument Options"="", "Flags"=0, "Help"="Sets selector repeated capability Component.\n\nAvailable Repeated Capabilities:\nNone\n\nRemote-control command(s):\n"}, {"Level"=2, "Class Only"=FALSE, "Identifier"="RSSCOPE_ATTR_DEEMBEDDING_COMPONENT_STATE", "Descriptive Name"="Deembedding Component State", "Data Type"=3, "Command"="DEEM{Channel}:COMP<Component>", "Access"=2, "Range Table"="", "Read Callback"="rsscope_FormatDeembeddingComponentRepCapBoolean_ReadCallback.vi", "Write Callback"="rsscope_FormatDeembeddingComponentRepCapBoolean_WriteCallback.vi", "Supported Models"="", "Instrument Options"="K121", "Flags"=0, "Help"="Enables or disables the indicated component for deembedding. The first and the last component are always enabled and cannot be disabled.\n\nAvailable Repeated Capabilities:\nChannel: CH1, CH2, CH3, CH4, CHExt\r\n\nRemote-control command(s):\nDEEMbedding<m>:COMPonent<n>[:STATe]"}, {"Level"=2, "Class Only"=FALSE, "Identifier"="RSSCOPE_ATTR_DEEMBEDDING_COMPONENT_TYPE", "Descriptive Name"="Deembedding Component Type", "Data Type"=0, "Command"="DEEM{Channel}:COMP<Component>:TYPE", "Access"=2, "Range Table"="RsScope_rngDeembedingComponentType", "Read Callback"="rsscope_FormatDeembeddingComponentRepCapInt32_ReadCallback.vi", "Write Callback"="rsscope_FormatDeembeddingComponentRepCapInt32_WriteCallback.vi", "Supported Models"="", "Instrument Options"="K121", "Flags"=0, "Help"="Sets the type of the indicated component. The first component is always DUT, the last component is PROBe or INPut.\n\nAvailable Repeated Capabilities:\nChannel: CH1, CH2, CH3, CH4, CHExt\r\n\nRemote-control command(s):\nDEEMbedding<m>:COMPonent<n>:TYPE"}, {"Level"=2, "Class Only"=FALSE, "Identifier"="RSSCOPE_ATTR_DEEMBEDDING_COMPONENT_NAME", "Descriptive Name"="Deembedding Component Name", "Data Type"=2, "Command"="DEEM{Channel}:COMP<Component>:NAME", "Access"=2, "Range Table"="", "Read Callback"="rsscope_FormatDeembeddingComponentRepCapString_ReadCallback.vi", "Write Callback"="rsscope_FormatDeembeddingComponentRepCapString_WriteCallback.vi", "Supported Models"="", "Instrument Options"="K121", "Flags"=0, "Help"="Sets a name for the indicated component that helps you identifying it.\n\nAvailable Repeated Capabilities:\nChannel: CH1, CH2, CH3, CH4, CHExt\r\n\nRemote-control command(s):\nDEEMbedding<m>:COMPonent<n>:NAME"}, {"Level"=2, "Class Only"=FALSE, "Identifier"="RSSCOPE_ATTR_DEEMBEDDING_COMPONENT_PORT_COUNT", "Descriptive Name"="Deembedding Component Port Count", "Data Type"=0, "Command"="DEEM{Channel}:COMP<Component>:PCO?", "Access"=0, "Range Table"="RsScope_rngDeembeddingComponentPort", "Read Callback"="rsscope_FormatDeembeddingComponentRepCapInt32_ReadCallback.vi", "Write Callback"="", "Supported Models"="", "Instrument Options"="K121", "Flags"=0, "Help"="Returns the number of all ports of the selected component (input ports and output ports). The number of ports depends on the attached probe. If a modular probe R&S RT-ZM or differential probe R&S& RT-ZD is used, the number of ports is 4. Otherwise, 2 ports are available.\n\nAvailable Repeated Capabilities:\nChannel: CH1, CH2, CH3, CH4, CHExt\r\n\nRemote-control command(s):\nDEEMbedding<m>:COMPonent<n>:PCOunt?"}, {"Level"=2, "Class Only"=FALSE, "Identifier"="RSSCOPE_ATTR_DEEMBEDDING_COMPONENT_MODE", "Descriptive Name"="Deembedding Component Mode", "Data Type"=0, "Command"="DEEM{Channel}:COMP<Component>:MODE", "Access"=2, "Range Table"="RsScope_rngDeembeddingComponentMode", "Read Callback"="rsscope_FormatDeembeddingComponentRepCapInt32_ReadCallback.vi", "Write Callback"="rsscope_FormatDeembeddingComponentRepCapInt32_WriteCallback.vi", "Supported Models"="", "Instrument Options"="K121", "Flags"=0, "Help"="Sets the probing mode.\n\nAvailable Repeated Capabilities:\nChannel: CH1, CH2, CH3, CH4, CHExt\r\n\nRemote-control command(s):\nDEEMbedding<m>:COMPonent<n>:MODE"}, {"Level"=2, "Class Only"=FALSE, "Identifier"="RSSCOPE_ATTR_DEEMBEDDING_COMPONENT_REMOVE_PROBE_LOADING", "Descriptive Name"="Deembedding Component Remove Probe Loading", "Data Type"=3, "Command"="DEEM{Channel}:COMP<Component>:LOAD:REMP", "Access"=2, "Range Table"="", "Read Callback"="rsscope_FormatDeembeddingComponentRepCapBoolean_ReadCallback.vi", "Write Callback"="rsscope_FormatDeembeddingComponentRepCapBoolean_WriteCallback.vi", "Supported Models"="", "Instrument Options"="K121", "Flags"=0, "Help"="Removes the loading of the probe if RSSCOPE_ATTR_DEEMBEDDING_COMPONENT_MODE is set to Probing. If the probe loading is removed, 
